vi "Modbus_Master.vi"() -> ()   [LabVIEW 2020]
uses:
  <vilib>/NI/Modbus Library/API/Wrapper/Create TCP Master.vi
  <vilib>/NI/Modbus Library/API/Master/Modbus Master.lvclass
  <vilib>/NI/Modbus Library/API/Wrapper/API Main.lvlib
panel:
  in  "Array":bool[](array[boolean])
  in  "address 2":u16
  in  "address":u16
  in  "stop":bool
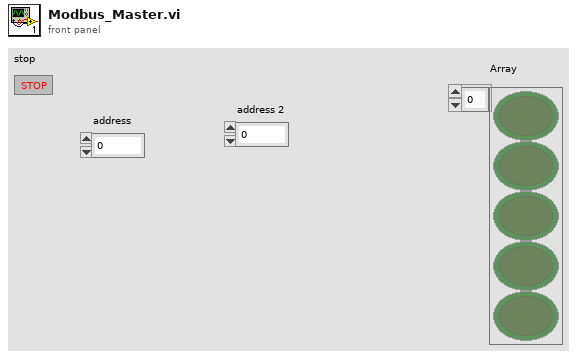
[diagram p1: front panel]
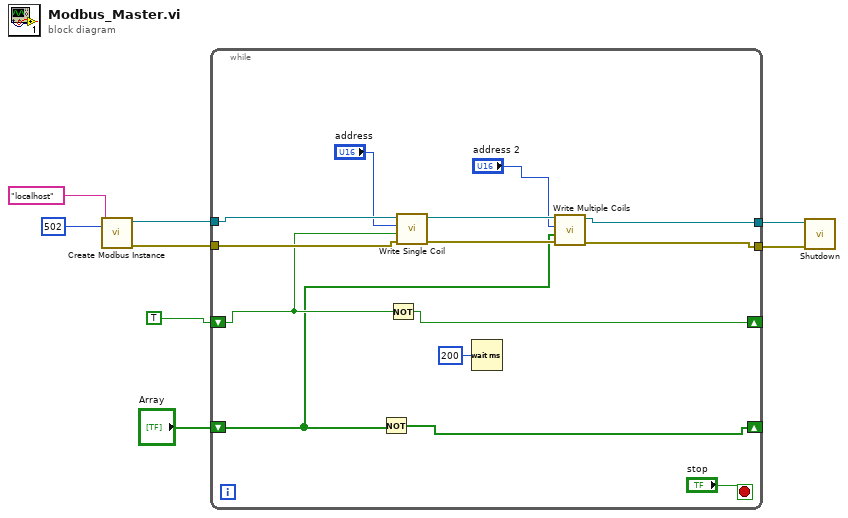
[diagram p0: block diagram]
diagram:
  n1 = call-poly <vilib>:"Create Modbus Instance.vi"("port (502)"=u16 502, "address"="localhost") -> ("error out"=w7:errorcluster, "TCP master instance"=w8:refnum<class "Modbus Master.lvclass">)  [unwired: 8 in]
  n2 = while {
    tunnel: w8 -> [w21]
    tunnel: w7 -> [w20]
    tunnel: [w13] -> w4
    tunnel: [w12] -> w3
    shift-right: [w17] -> _
    shift-left: TRUE -> [w16]
    shift-right: [w10] -> _
    shift-left: "Array" -> [w9]
    stop <- "stop" stop-if-true
    n3 = Not(x=w9) -> (.not. x?=w10:bool[])
    n4 = Not(x=w16) -> (.not. x?=w17:bool)
    n5 = call-dynamic "Write Single Coil.vi"("error in"=w20, "coil to write"=w16, "address"="address", "Modbus master in"=w21) -> ("error out"=w14:errorcluster, "Modbus master out"=w15:refnum<class "Modbus Master.lvclass">)  [unwired: 6 in]
    n6 = Wait (ms)(milliseconds to wait=u32 200) -> ()  [unwired: 1 out]
    n7 = call-dynamic "Write Multiple Coils.vi"("error in"=w14, "coils to write"=w9, "starting address"="address 2", "Modbus master in"=w15) -> ("error out"=w12:errorcluster, "Modbus master out"=w13:refnum<class "Modbus Master.lvclass">)  [unwired: 6 in]
  }
  n8 = call-dynamic "Shutdown.vi"("error in"=w3, "Modbus master in"=w4) -> ()  [unwired: 9 in, 1 out]
